vi "AlliGator Load HDF5 FLI Dataset Prelude.vi"(8 "error in (no error)":errorcluster, 11 "File Path":path) -> (0 "error out":errorcluster, 1 "Metadata":string, 2 "FLI Data File Information":T1, 3 "File Path out":path, 4 "Data Description":string)   [LabVIEW 2021, in "AlliGator HDF5.lvlib"]
doc: "Initial steps of loading a HDF5 FLI dataset file."
uses:
  AlliGator HDF5.lvlib
  AlliGator FLI Data File Information.ctl
  Phasor/Phasor Fluorescence Lifetime Parameters v3.ctl
  AlliGator FLI Dataset Type.ctl
  AlliGator Files.lvlib
  Phasor/Phasor.lvlib
panel:
  # "see the AlliGator License on the block diagram (Ctrl+E or Window:Show Block Diagram)"
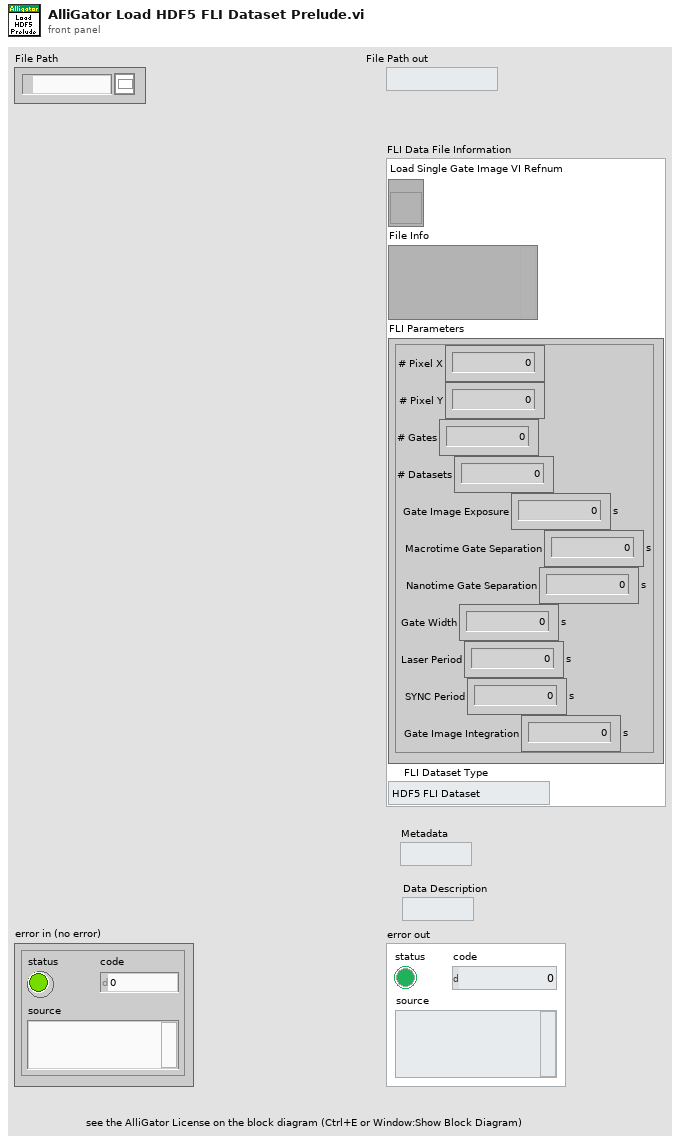
[diagram p1: front panel]
types:
  T1 = typedef "AlliGator HDF5.lvlib/AlliGator FLI Data File Information.ctl" = cluster{"Load Single Gate Image VI Refnum":refnum<vi>, "File Info":variant, "FLI Parameters":T2, "FLI Dataset Type":T3}
  T2 = typedef "Phasor.lvlib/Phasor Fluorescence Lifetime Parameters v3.ctl" = cluster{"# Pixel X":i32, "# Pixel Y":i32, "# Gates":i32, "# Datasets":i32, "Gate Image Exposure":dbl[unit], "Macrotime Gate Separation":dbl[unit], "Nanotime Gate Separation":dbl[unit], "Gate Width":dbl[unit], "Laser Period":dbl[unit], "SYNC Period":dbl[unit], "Gate Image Integration":dbl[unit]}
  T3 = typedef "AlliGator Files.lvlib/AlliGator FLI Dataset Type.ctl" = enum16{"HDF5 FLI Dataset", "Gate Image Folder", ".sdt FLI Dataset (Becker & Hickl)", ".ptu FLI Dataset (PicoQuant)", "SS1 FLI Dataset", "SS2 FLI Dataset", "I/m/phi Dataset", ".bin FLI Dataset (PicoQuant Binned)", ".bin FLI Dataset (Piccolo Binned)"}
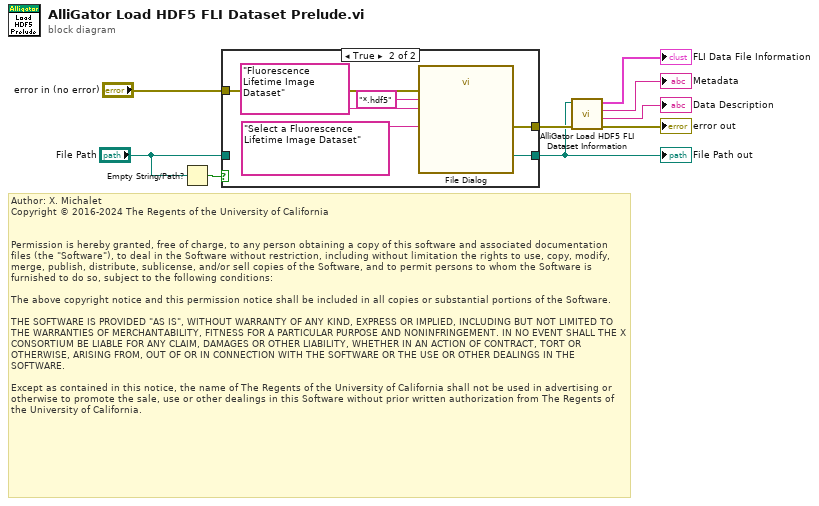
[diagram p0: block diagram]
diagram:
  # "Author: X. Michalet\nCopyright © 2016-2024 The Regents of the University of California\n \n\nPermission is hereby granted, free of charge, to any person obtaining a copy of this software and associated documentation files (the \"Software\"), to deal in the Software without restriction, including without limitation the rights to use, copy, modify, merge, publish, distribute, sublicense, and/or sell copies of the Software, and to permit persons to whom the Software is furnished to do so, subject to the following conditions:\n\nThe above copyright notice and this permission notice shall be included in all copies or substantial portions of the Software.\n\nTHE SOFTWARE IS PROVIDED \"AS IS\", WITHOUT WARRANTY OF ANY KIND, EXPRESS OR IMPLIED, INCLUDING BUT NOT LIMITED TO THE WARRANTIES OF MERCHANTABILITY, FITNESS FOR A PARTICULAR PURPOSE AND NONINFRINGEMENT. IN NO EVENT SHALL THE X CONSORTIUM BE LIABLE FOR ANY CLAIM, DAMAGES OR OTHER LIABILITY, WHETHER IN AN ACTION OF CONTRACT, TORT OR OTHERWISE, ARISING FROM, OUT OF OR IN CONNECTION WITH THE SOFTWARE OR THE USE OR OTHER DEALINGS IN THE SOFTWARE.\n\nExcept as contained in this notice, the name of The Regents of the University of California shall not be used in advertising or otherwise to promote the sale, use or other dealings in this Software without prior written authorization from The Regents of the University of California."
  n1 = Empty String/Path?(string/path="File Path") -> (empty?=w3:bool)
  n2 = case shown="True" w3 {
    tunnel: "error in (no error)" -> [w10 w17]
    tunnel: [w11 w13] -> w4
    tunnel: [w10 w12] -> w5
    tunnel: "File Path" -> [w11 _]
    frame False {
    }
    frame True {
      n3 = call "File Dialog"("prompt"="Select a Fluorescence Lifetime Image Dataset", "error in"=w17, "pattern (all files)"="*.hdf5", "pattern label"="Fluorescence Lifetime Image Dataset") -> ("selected path"=w13:path, "error out"=w12:errorcluster)  [unwired: 8 in, 2 out]
    }
  }
  "File Path out" <- w4
  n4 = call "AlliGator Load HDF5 FLI Dataset Information.vi"("Error In"=w5, "File Path"=w4) -> ("error out"=→"error out":errorcluster, "Data Description"=→"Data Description":string, "Metadata"=→"Metadata":string, "FLI Data File Information"=→"FLI Data File Information":T1)  [unwired: 5 in, 1 out]
